vi "RollerSoftStart.vi"(8 "error in (no error)":errorcluster, 11 "milliseconds to wait":u32=500) -> (0 "error out":errorcluster)   [LabVIEW 2013]
uses:
  PickupSoftStartStates.ctl
  <vilib>/Rock Robotics/WPI/Solenoid/WPI_SolenoidValue.ctl
  <vilib>/Rock Robotics/WPI/Solenoid/WPI_SolenoidSetEnum.vi
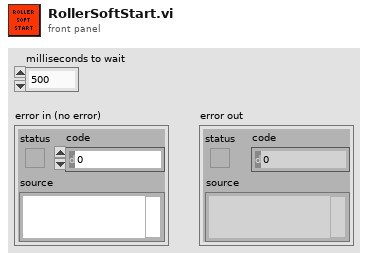
[diagram p1: front panel]
types:
  T1 = typedef "PickupSoftStartStates.ctl" = enum16{"Start Rollers", "Wait", "Deploy"}
  T2 = typedef "WPI_SolenoidValue.ctl" = enum16{"Off", "On", "Forward", "Reverse"}
  T3 = typedef "WPI_MotorControlDeviceRef.ctl" = cluster{"DeviceStatus":errorcluster, "Type":enum16{"PWM", "CAN"}, "PWM":cluster{"Digital Module":T4, "PWM Channel":T5, "DeadBand":T6}, "CAN":cluster{"Device Number":u8, "Control Mode":T7, "Semaphore":T8, "Max Vout":dbl}, "Invert":bool, "TransformRef":T9, "InvTransformRef":T9}
  T4 = typedef "FPGA_TypedefDigitalModule.ctl" = enum16{"Digital Module 1", "Digital Module 2"}
  T5 = typedef "FPGA_DIOPWMChannel.ctl" = enum8{"PWM 1", "PWM 2", "PWM 3", "PWM 4", "PWM 5", "PWM 6", "PWM 7", "PWM 8", "PWM 9", "PWM 10", "Invalid"}
  T6 = typedef "WPI_PWMDeadband.ctl" = cluster{"Name":string, "maxPositivePwm":i32, "minPositivePwm":i32, "centerPwm":i32, "maxNegativePwm":i32, "minNegativePwm":i32, "angularRange":u16}
  T7 = typedef "WPI_CANJaguar_ControlMode.ctl" = enum8{"Percent VBus", "Current", "Speed", "Position", "Voltage"}
  T8 = typedef "Semaphore RefNum" = refnum<k1>
  T9 = typedef "WPI_PWMTransform_ConPane.ctl" = refnum<vi>
  T10 = typedef "WPI_SolenoidDevRef.ctl" = cluster{"DevStatus":errorcluster, "Solenoid Module":T11, "Forward Solenoid Channel":T12, "Reverse Solenoid Channel":T12}
  T11 = typedef "FPGA_TypedefSolenoidModule.ctl" = enum16{"Solenoid Module 1", "Solenoid Module 2"}
  T12 = typedef "WPI_SolenoidChannel.ctl" = enum8{"Solenoid 1", "Solenoid 2", "Solenoid 3", "Solenoid 4", "Solenoid 5", "Solenoid 6", "Solenoid 7", "Solenoid 8", "Invalid"}
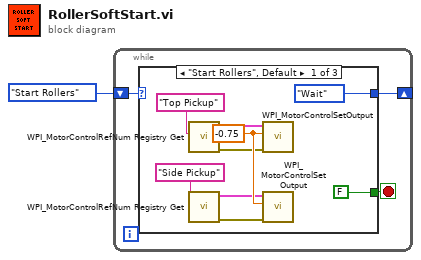
[diagram p0: block diagram]
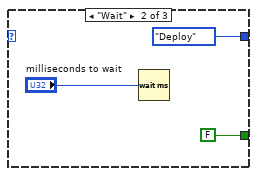
[diagram p2: hidden frame]
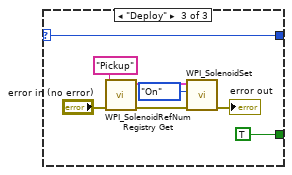
[diagram p3: hidden frame]
diagram:
  n1 = while {
    shift-right: [w3] -> _
    shift-left: PickupSoftStartStates."Start Rollers" -> [w4]
    stop <- w2 stop-if-true
    n2 = case shown="\"Start Rollers\", Default" w4 {
      selector: w4 -> [_ _ w20]
      tunnel: [PickupSoftStartStates."Wait" PickupSoftStartStates."Deploy" w20] -> w3
      tunnel: [FALSE FALSE TRUE] -> w2
      frame "Start Rollers", Default {
        w13 = -0.75 ("Output")
        n3 = call <vilib>:"WPI_MotorControlRefNum Registry Get.vi"("refnum name"="Top Pickup") -> ("error out"=w11:errorcluster, "MotorControlDevRef"=w7:T3)  [unwired: 9 in]
        n4 = call <vilib>:"WPI_MotorControlRefNum Registry Get.vi"("refnum name"="Side Pickup") -> ("error out"=w9:errorcluster, "MotorControlDevRef"=w10:T3)  [unwired: 9 in]
        n5 = call <vilib>:"WPI_MotorControlSetOutput.vi"("error in (no error)"=w11, "Output"=w13, "MotorControlDevRef"=w7) -> ()  [unwired: 6 in, 3 out]
        n6 = call <vilib>:"WPI_MotorControlSetOutput.vi"("error in (no error)"=w9, "Output"=w13, "MotorControlDevRef"=w10) -> ()  [unwired: 6 in, 3 out]
      }
      frame "Wait" {
        n7 = Wait (ms)(milliseconds to wait="milliseconds to wait") -> ()  [unwired: 1 out]
      }
      frame "Deploy" {
        n8 = call <vilib>:"WPI_SolenoidRefNum Registry Get.vi"("error in (no error)"="error in (no error)", "refnum name"="Pickup") -> ("error out"=w22:errorcluster, "SolenoidDevRef"=w23:T10)  [unwired: 8 in]
        n9 = call-poly <vilib>:"WPI_SolenoidSet.vi"("error in (no error)"=w22, "Value"=WPI_SolenoidValue."On", "SolenoidDevRef"=w23) -> ("error out"=→"error out":errorcluster)  [unwired: 7 in, 1 out]
      }
    }
  }
